vi "期末11.vi"() -> ()   [LabVIEW 2014]
uses:
  <vilib>/vision/NI_Vision_Development_Module.lvlib
panel:
  out "output array":dbl[](array[numeric])
  out "x/y":dbl
  out "Image Out 2":T1(plugin-control)
  out "ROI":T2
  in  "紀錄中點座標和":bool
  out "填入飽和磁場分量尖點座標和 2":dbl
  in  "3. Number of Erosion":i32=10
  out "Image Out":T1(plugin-control)
  in  "紀錄電流":dbl[](array[numeric])
  in  "Tab Control 2":enum32{"座標", "座標和", "作圖"}(tab)
  out "瞬間尖點座標":dbl[][](array[numeric])
  out "尖點座標和":dbl[](array[numeric])
  out "相減結果":dbl[](array[numeric])
  out "分量-電流":cluster{"紀錄電流":dbl[], dbl[]}(graph)
  in  "紀錄":bool
  in  "結束實驗":bool
  in  "1. 範圍選擇":T3={"色相（H）"={0, 255}, "飽和度（S）"={0, 255}, "亮度（L）"={0, 255}} {"亮度（L）" scale=0.0..255.0; "飽和度（S）" scale=0.0..255.0; "色相（H）" scale=0.0..255.0}
  out "Number of Particles":i32
  out "output cluster":cluster{"X":dbl, "Y":dbl}
  in  "Tab Control":T4(tab)
  out "1. 顏色選取":T1(plugin-control)
  out "2. 填補空隙":T1(plugin-control)
  out "3. 移除雜點":T1(plugin-control)
  out "4. 形狀修正":T1(plugin-control)
  out "5. 選取結果":T1(plugin-control)
  out "Particle Measurements":dbl[][](array[numeric])
  out "Error Out":errorcluster
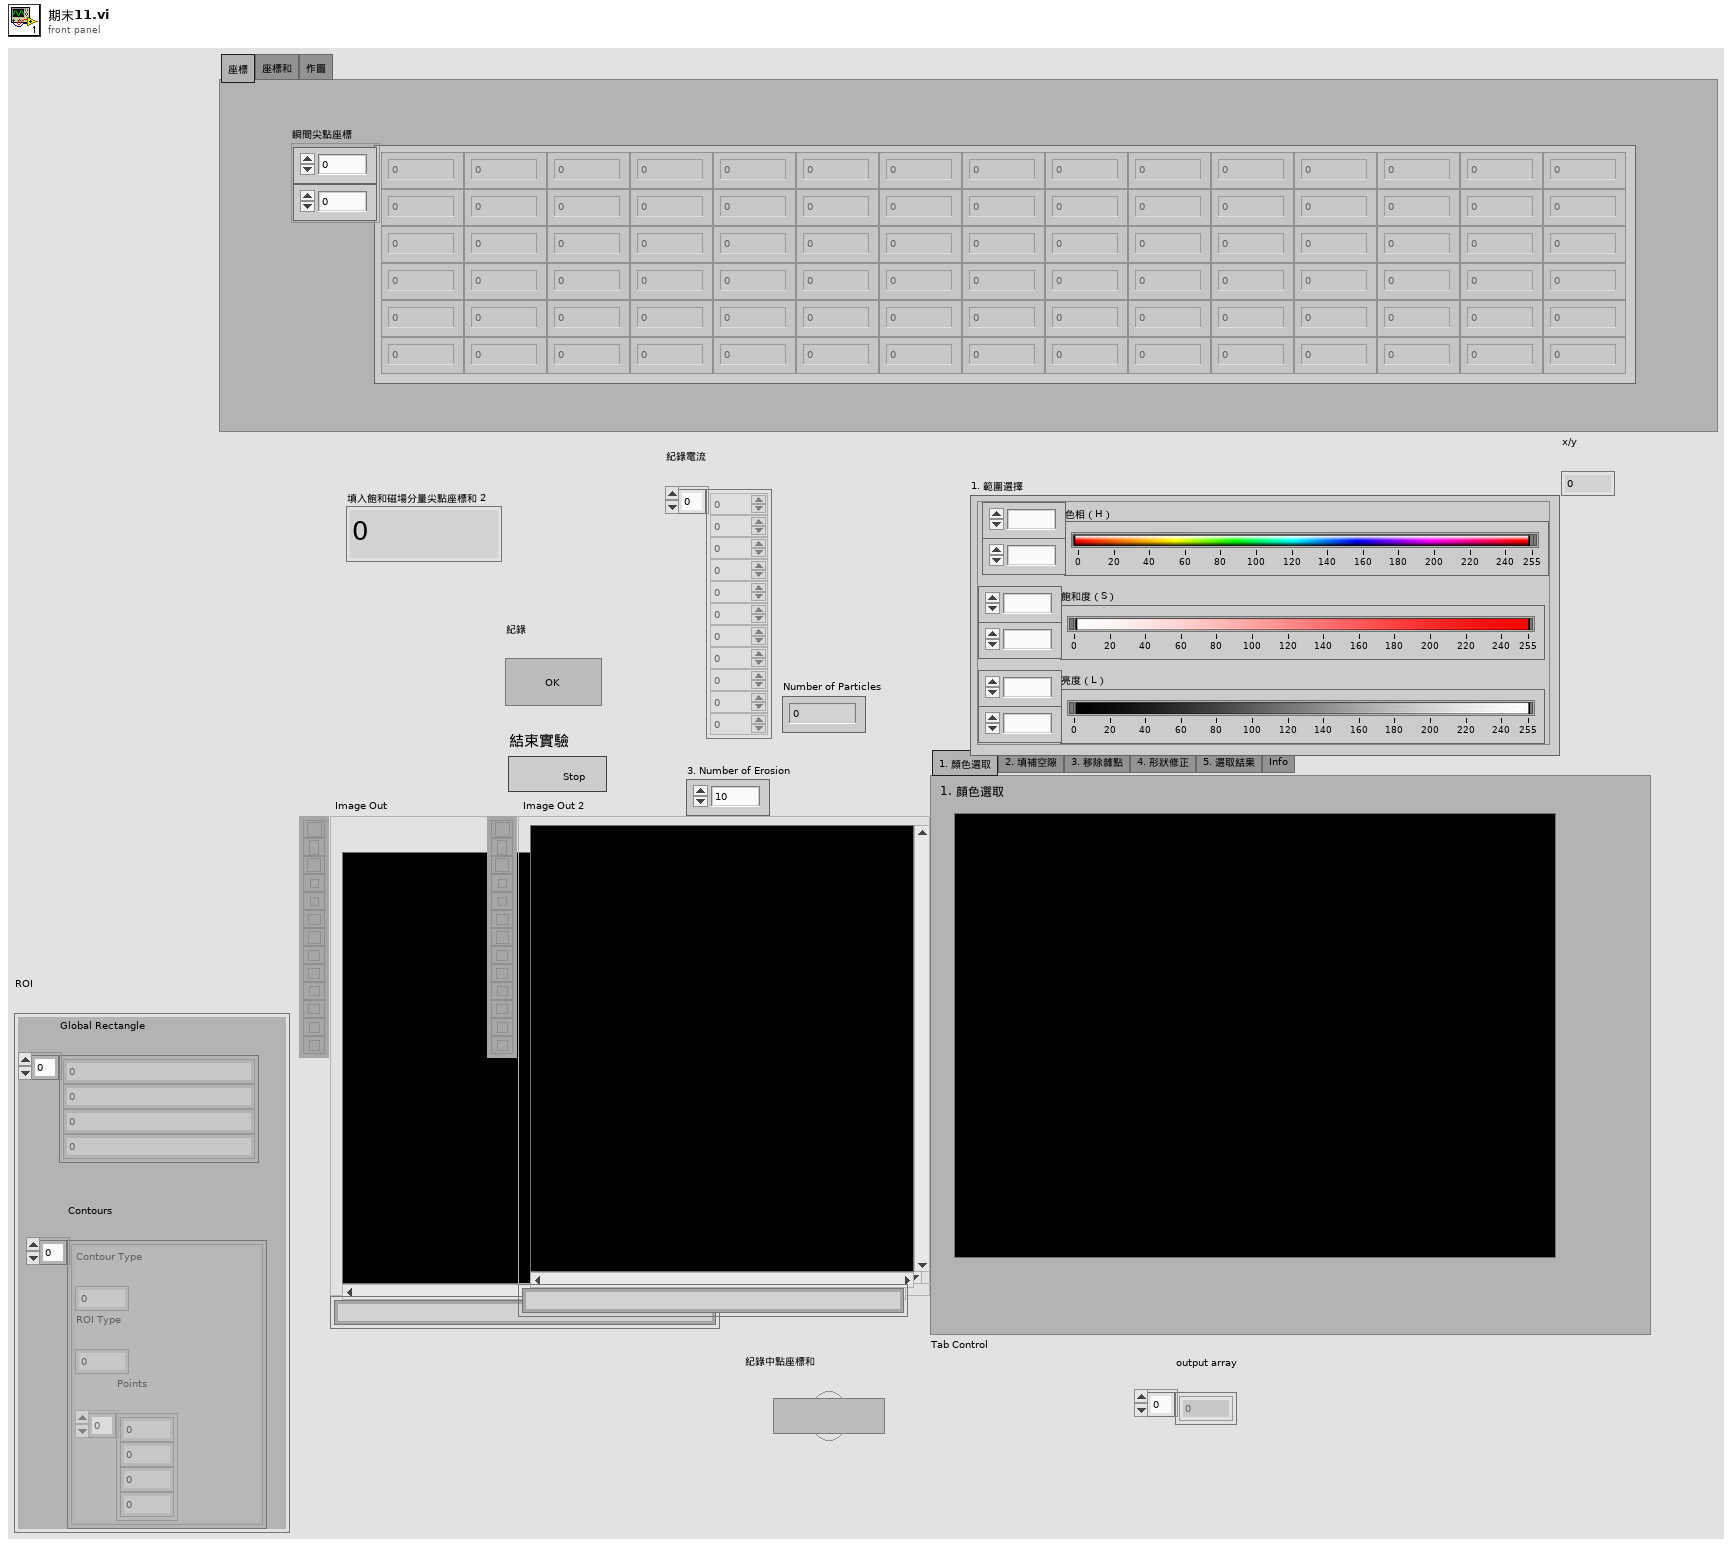
[diagram p1: front panel]
types:
  T1 = typedef "IMAQ Image.ctl" = refnum<image>
  T2 = cluster{"Global Rectangle":i32[], "Contours":cluster{"Contour Type":u32, "ROI Type":u32, "Points":i32[]}[]}
  T3 = cluster{"色相（H）":cluster{u8, u8}, "飽和度（S）":cluster{u8, u8}, "亮度（L）":cluster{u8, u8}}
  T4 = enum32{"1. 顏色選取", "2. 填補空隙", "3. 移除雜點", "4. 形狀修正", "5. 選取結果", "Info"}
  T5 = typedef "Image Type" = u32
  T6 = cluster{"Numeric":dbl, "Numeric":dbl, "Numeric":dbl, "Numeric":dbl}
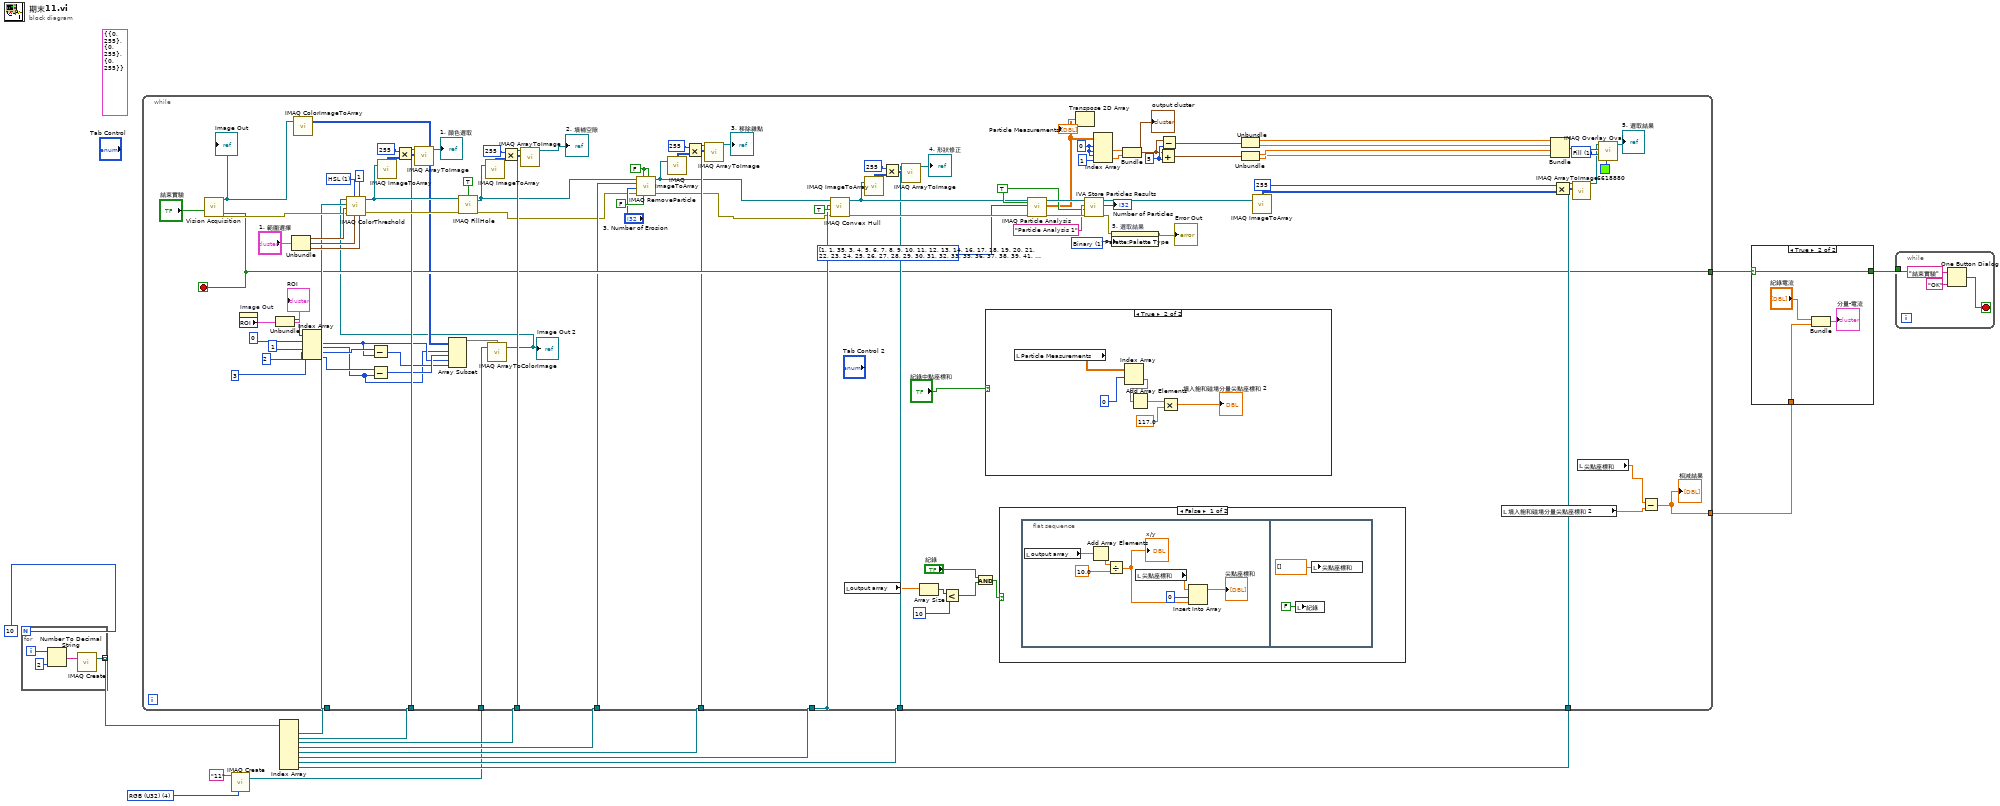
[diagram p0: block diagram]
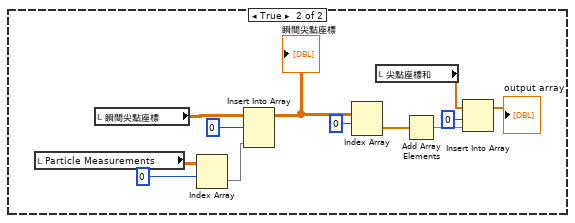
[diagram p3: hidden frame]
diagram:
  w3 = T5 4 items=["Grayscale (U8)", "Grayscale (I16)", "Grayscale (SGL)", "Complex (CSG)", "RGB (U32)", "HSL (U32)", "RGB (U64)", "Grayscale (U16)"] ("Image Type")
  (unwired) T3 {"色相（H）"={0, 255}, "飽和度（S）"={0, 255}, "亮度（L）"={0, 255}} ("範圍選擇")
  n1 = for {
    N: 10 -> [_]
    tunnel: [w17] -> w16 mode=indexing
    i -> [w19]
    n2 = Number To Decimal String(number=w19, width (-)=2) -> (decimal integer string=w18:string)
    n3 = call "IMAQ Create"("Image Name"=w18) -> ("New Image"=w17:T1)  [unwired: 4 in, 1 out]
  }
  n4 = call "IMAQ Create"("Image Name"="11", "Image Type"=w3) -> ("New Image"=w4:T1)  [unwired: 3 in, 1 out]
  n5 = Index Array(array=w16) -> (element #1=w15:T1, element #2=w14:T1, element #3=w13:T1, element #4=w6:T1, element #5=w5:T1, element #6=w11:T1, element #7=w10:T1, element #8=w9:T1)  [unwired: 8 in]
  n6 = while {
    tunnel: w13 -> [w95]
    tunnel: w11 -> [w106]
    tunnel: [w106] -> _
    tunnel: w14 -> [w100]
    tunnel: w15 -> [w94]
    tunnel: w10 -> [w88]
    tunnel: w9 -> [w65]
    tunnel: [w61] -> w8
    tunnel: [w21] -> w7
    tunnel: w6 -> [w54]
    tunnel: w5 -> [w53]
    tunnel: w4 -> [w38]
    stop <- w61 stop-if-true
    w58 = FALSE ("Connectivity 4/8 (8)")
    w70 = u32 1 items=["Frame", "Fill"] ("Drawing Mode (Frame)")
    w79 = 5
    w84 = 0
    w108 = u32 1 items=["Grayscale", "Binary", "Gradient", "Rainbow", "Temperature", "User Defined"] ("Palette")
    w113 = i32[] [1, 1, 35, 3, 4, 5, 6, 7, 8, 9, 10, 11, 12, 13, 14, 16, 17, 18, 19, 20, 21, 22, 23, 24, 25, 26, 27, 28, 29, 30, 31, 32, 33, 35, 36, 37, 38, 39, 41, 42, 43, 45, 46, 48, 49, 50, 51, 53, 54, 55, 56, 58, 59, 60, 61, 62, 63, 64, 65, 66, 68, 69, 70, 71, 72, 73, 74, 75, 76, 77, 78, 79, 80, 81, 82, 83, 84, 85, 86, 87, 88] items=["Center of Mass X", "Center of Mass Y", "First Pixel X", "First Pixel Y", "Bounding Rect Left", "Bounding Rect Top", "Bounding Rect Right", "Bounding Rect Bottom", "Max Feret Diameter Start X", "Max Feret Diameter Start Y", "Max Feret Diameter End X", "Max Feret Diameter End Y", "Max Horiz. Segment Length Left", "Max Horiz. Segment Length Right", "Max Horiz. Segment Length Row", "-", "Bounding Rect Width", "Bounding Rect Height", "Bounding Rect Diagonal", "Perimeter", "Convex Hull Perimeter", "Holes' Perimeter", "Max Feret Diameter", "Equivalent Ellipse Major Axis", "Equivalent Ellipse Minor Axis", "Equivalent Ellipse Minor Axis (Feret)", "Equivalent Rect Long Side", "Equivalent Rect Short Side", "Equivalent Rect Diagonal", "Equivalent Rect Short Side (Feret)", "Average Horiz. Segment Length", "Average Vert. Segment Length", "Hydraulic Radius", "Waddel Disk Diameter", "-", "Area", "Holes' Area", "Particle & Holes' Area", "Convex Hull Area", "Image Area", "-", "Number of Holes", "Number of Horiz. Segments", "Number of Vert. Segments", "-", "Orientation", "Max Feret Diameter Orientation", "-", "% Area/Image Area", "% Area/(Particle & Holes' Area)", "Ratio of Equivalent Ellipse Axes", "Ratio of Equivalent Rect Sides", "-", "Elongation Factor", "Compactness Factor", "Heywood Circularity Factor", "Type Factor", "-", "Sum X", "Sum Y", "Sum XX", "Sum XY", "Sum YY", "Sum XXX", "Sum XXY", "Sum XYY", "Sum YYY", "-", "Moment of Inertia XX", "Moment of Inertia XY", "Moment of Inertia YY", "Moment of Inertia XXX", "Moment of Inertia XXY", "Moment of Inertia XYY", "Moment of Inertia YYY", "Norm. Moment of Inertia XX", "Norm. Moment of Inertia XY", "Norm. Moment of Inertia YY", "Norm. Moment of Inertia XXX", "Norm. Moment of Inertia XXY", "Norm. Moment of Inertia XYY", "Norm. Moment of Inertia YYY", "Hu Moment 1", "Hu Moment 2", "Hu Moment 3", "Hu Moment 4", "Hu Moment 5", "Hu Moment 6", "Hu Moment 7"] ("Pixel Measurements")
    w115 = TRUE ("Connectivity 4/8 (8)")
    w124 = u16 1 items=["RGB", "HSL", "HSV", "HSI"] ("Color Mode")
    n7 = call "Vision Acquisition"("Stop (F)"="結束實驗") -> ("Image Out"=w46:T1, "Stopped"=w61:bool, "error out"=w119:errorcluster)  [unwired: 24 in]
    "Image Out" <- w46
    n8 = property on="Image Out" class="ImageControl"() -> ("ROI"=w44:T2)  [unwired: 2 in, 2 out]
    "ROI" <- w44
    n9 = Unbundle(w44) -> ("Global Rectangle"=w43:i32[])  [unwired: 1 out]
    n10 = Unbundle("1. 範圍選擇") -> ("色相（H）"=w123:cluster{u8, u8}, "飽和度（S）"=w122:cluster{u8, u8}, "亮度（L）"=w121:cluster{u8, u8})
    n11 = call "IMAQ ColorImageToArray"("Image"=w46) -> ("Image Pixels (U32)"=w45:u32[][])  [unwired: 3 in, 2 out]
    n12 = Index Array(array=w43, index #1=0 ("index"), index #2=1 ("index"), index #3=2 ("index"), index #4=3 ("index")) -> (element #1=w33:i32, element #2=w31:i32, element #3=w36:i32, element #4=w32:i32)
    n13 = Subtract(x=w36, y=w33) -> (x-y=w34:i32)
    n14 = Subtract(x=w32, y=w31) -> (x-y=w35:i32)
    n15 = Array Subset(array=w45, index (row)=w31, length (row)=w35, index (col)=w33, length (col)=w34) -> (w37:u32[][])
    n16 = call "IMAQ ArrayToColorImage"("Image Pixels (U32)"=w37, "Image"=w38) -> ("Image Out"=w30:T1)  [unwired: 3 in, 1 out]
    "Image Out 2" <- w30
    n17 = call "IMAQ ColorThreshold"("Blue or Luma or Val or Inten Range"=w121, "Replace Value"=1, "Green or Sat Range"=w122, "Color Mode"=w124, "error in (no error)"=w119, "Red or Hue Range"=w123, "Image Dst"=w94, "Image Src"=w30) -> ("error out"=w110:errorcluster, "Image Dst Out"=w105:T1)  [unwired: 2 out]
    n18 = call "IMAQ ImageToArray"("Image"=w105) -> ("Image Pixels (U8)"=w103:u8[][])  [unwired: 3 in, 4 out]
    n19 = Multiply(x=255, y=w103) -> (x*y=w102:i32[][])
    n20 = call "IMAQ ArrayToImage"("Image Pixels (U8)"=w102, "Image"=w100) -> ("Image Out"=→"1. 顏色選取":T1)  [unwired: 8 in, 1 out]
    n21 = call "IMAQ FillHole"("error in (no error)"=w110, "Image Src"=w105, "Connectivity 4/8 (8)"=TRUE) -> ("error out"=w52:errorcluster, "Image Dst Out"=w50:T1)  [unwired: 1 in, 2 out]
    n22 = call "IMAQ ImageToArray"("Image"=w50) -> ("Image Pixels (U8)"=w98:u8[][])  [unwired: 3 in, 4 out]
    n23 = Multiply(x=255, y=w98) -> (x*y=w99:i32[][])
    n24 = call "IMAQ ArrayToImage"("Image Pixels (U8)"=w99, "Image"=w95) -> ("Image Out"=→"2. 填補空隙":T1)  [unwired: 8 in, 1 out]
    n25 = call "IMAQ RemoveParticle"("Connectivity 4/8 (8)"=w58, "Low Pass/High Pass (Low)"=FALSE, "Square/Hexa (Square)"=w58, "error in (no error)"=w52, "Number of Erosion"="3. Number of Erosion", "Image Dst"=w54, "Image Src"=w50) -> ("error out"=w51:errorcluster, "Image Dst Out"=w49:T1)  [unwired: 3 out]
    n26 = call "IMAQ ImageToArray"("Image"=w49) -> ("Image Pixels (U8)"=w48:u8[][])  [unwired: 3 in, 4 out]
    n27 = Multiply(x=255, y=w48) -> (x*y=w56:i32[][])
    n28 = call "IMAQ ArrayToImage"("Image Pixels (U8)"=w56, "Image"=w53) -> ("Image Out"=→"3. 移除雜點":T1)  [unwired: 8 in, 1 out]
    n29 = call "IMAQ Convex Hull"("error in (no error)"=w51, "Connectivity 4/8 (8)"=TRUE, "Image Dst"=w106, "Image Src"=w49) -> ("error out"=w114:errorcluster, "Image Dst Out"=w89:T1)  [unwired: 6 out]
    n30 = local read "output array"() -> (w24:dbl[])
    n31 = call "IMAQ ImageToArray"("Image"=w89) -> ("Image Pixels (U8)"=w92:u8[][])  [unwired: 3 in, 4 out]
    n32 = Multiply(x=255, y=w92) -> (x*y=w93:i32[][])
    n33 = call "IMAQ ArrayToImage"("Image Pixels (U8)"=w93, "Image"=w88) -> ("Image Out"=→"4. 形狀修正":T1)  [unwired: 8 in, 1 out]
    n34 = Array Size(array=w24) -> (size(s)=w28:i32)
    n35 = Less?(x=w28, y=10) -> (x < y?=w26:bool)
    n36 = And(x="紀錄", y=w26) -> (x .and. y?=w25:bool)
    n37 = case shown="True" "紀錄中點座標和" {
      frame False {
      }
      frame True {
        n38 = local read "Particle Measurements"() -> (w151:dbl[][])
        n39 = Index Array(array=w151, index (row)=0) -> (element=w150:dbl[])  [unwired: 1 in]
        n40 = Add Array Elements(numeric array=w150) -> (sum=w149:dbl)
        n41 = Multiply(x=w149, y=117.0) -> (x*y=→"填入飽和磁場分量尖點座標和 2":dbl)
      }
    }
    n42 = case shown="False" w25 {
      frame False {
        n43 = flat-sequence {
          frame #0 {
            n44 = local read "output array"() -> (w131:dbl[])
            n45 = Add Array Elements(numeric array=w131) -> (sum=w132:dbl)
            n46 = Divide(x=w132, y=10.0) -> (x/y=w128:dbl)
            "x/y" <- w128
            n47 = local read "尖點座標和"() -> (w130:dbl[])
            n48 = Insert Into Array(array=w130, index=0, new element=w128) -> (→"尖點座標和":dbl[])
          }
          frame #1 {
            n49 = local write "紀錄"(FALSE ("紀錄")) -> ()
            n50 = local write "尖點座標和"(dbl[] [] ("尖點座標和")) -> ()
          }
        }
      }
      frame True {
        n51 = local read "Particle Measurements"() -> (w137:dbl[][])
        n52 = local read "瞬間尖點座標"() -> (w142:dbl[][])
        n53 = Index Array(array=w137, index (row)=0) -> (element=w141:dbl[])  [unwired: 1 in]
        n54 = Insert Into Array(array=w142, index (row)=0 ("index"), new element=w141) -> (w144:dbl[][])  [unwired: 1 in]
        "瞬間尖點座標" <- w144
        n55 = Index Array(array=w144, index (row)=0) -> (element=w146:dbl[])  [unwired: 1 in]
        n56 = local read "尖點座標和"() -> (w138:dbl[])
        n57 = Add Array Elements(numeric array=w146) -> (sum=w140:dbl)
        n58 = Insert Into Array(array=w138, index=0 ("index (row)"), new element=w140) -> (→"output array":dbl[])
      }
    }
    n59 = call "IMAQ Particle Analysis"("Connectivity 4/8 (8)"=w115, "error in (no error)"=w114, "Pixel Measurements"=w113, "Image"=w89) -> ("error out"=w118:errorcluster, "Particle Measurements (Pixels)"=w85:dbl[][], "Image Out (duplicate)"=w116:T1)  [unwired: 1 in, 4 out]
    n60 = Transpose 2D Array(2D array=w85) -> (transposed array=→"Particle Measurements":dbl[][])
    n61 = call <vilib>:"IVA Store Particles Results.vi"("error in (no error)"=w118, "Connectivity 4/8 (8)"=w115, "Step Name"="Particle Analysis 1", "Image in"=w116) -> ("error out"=w109:errorcluster, "Number of Particles"=→"Number of Particles":i32, "Image dup"=w69:T1)  [unwired: 5 out]
    n62 = Index Array(array=w85, index (row) #1=w84, index (col) #1=w84, index (row) #2=w84, index (col) #2=1) -> (element #1=w82:dbl, element #2=w81:dbl)
    n63 = property on="5. 選取結果" class="ImageControl"(error in=w109, "Palette:Palette Type"=w108) -> (error out=→"Error Out":errorcluster)  [unwired: 1 in, 1 out]
    n64 = Bundle("Numeric"=w82, "Numeric"=w81) -> (w78:cluster{"Numeric":dbl, "Numeric":dbl})  [unwired: 1 in]
    "output cluster" <- w78
    n65 = Add(x=w78, y=w79) -> (x+y=w76:cluster{"Numeric":dbl, "Numeric":dbl})
    n66 = Subtract(x=w78, y=w79) -> (x-y=w77:cluster{"Numeric":dbl, "Numeric":dbl})
    n67 = Unbundle(w77) -> ("Numeric"=w75:dbl, "Numeric"=w74:dbl)
    n68 = Unbundle(w76) -> ("Numeric"=w73:dbl, "Numeric"=w72:dbl)
    n69 = call "IMAQ ImageToArray"("Image"=w69) -> ("Image Pixels (U8)"=w66:u8[][])  [unwired: 3 in, 4 out]
    n70 = local read "填入飽和磁場分量尖點座標和 2"() -> (w22:dbl)
    n71 = Bundle("Numeric"=w75, "Numeric"=w74, "Numeric"=w73, "Numeric"=w72) -> (w71:T6)  [unwired: 1 in]
    n72 = Multiply(x=255, y=w66) -> (x*y=w67:i32[][])
    n73 = call "IMAQ ArrayToImage"("Image Pixels (U8)"=w67, "Image"=w65) -> ("Image Out"=w64:T1)  [unwired: 8 in, 1 out]
    n74 = local read "尖點座標和"() -> (w23:dbl[])
    n75 = call "IMAQ Overlay Oval"("Color"=u32 6618880, "Drawing Mode (Frame)"=w70, "Bounding Rectangle"=w71, "Image"=w64) -> ("Image Out"=→"5. 選取結果":T1)  [unwired: 6 in, 1 out]
    n76 = Subtract(x=w23, y=w22) -> (x-y=w21:dbl[])
    "相減結果" <- w21
  }
  n77 = case shown="True" w8 {
    selector: w8 -> [w153 w157]
    tunnel: [w153 w157] -> w1
    tunnel: w7 -> [_ w156]
    frame False {
    }
    frame True {
      n78 = Bundle("紀錄電流"="紀錄電流", w156) -> (→"分量-電流":cluster{"紀錄電流":dbl[], dbl[]})  [unwired: 1 in]
    }
  }
  n79 = while {
    tunnel: w1 -> [_]
    stop <- w160 stop-if-true
    n80 = One Button Dialog(message="結束實驗", button name ("OK")="OK") -> (true=w160:bool)
  }
